vi "RIOduino Periodic.vi"() -> (3 "GearMode":string)   [LabVIEW 2016]
uses:
  TypeDefs/GearCollectState_Type.ctl
  TypeDefs/TurretAimState_Type.ctl
  Global_Var-RefNum/GlobalVar_LED.vi
  <vilib>/Rock Robotics/SystemInterfaces/i2clib/i2c_bus.ctl
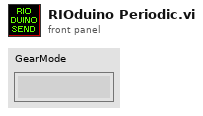
[diagram p1: front panel]
types:
  T1 = typedef "TurretAimState_Type.ctl" = enum16{"Idle", "SearchLeft", "SearchRight", "FindNewTarget", "TargetAcquired"}
  T2 = typedef "GearCollectState_Type.ctl" = enum16{"Store Gear", "Wait For Gear", "Idle"}
  T3 = typedef "i2c_bus.ctl" = enum16{"I2C On-Board", "I2C MXP", "Invalid"}
  T4 = typedef "WPI_I2CDevRef.ctl" = cluster{"DevStatus":errorcluster, "Device Address":u8, "Handle":i32, "I2C Bus":T3}
  T5 = typedef "GearPlaceState_Type.ctl" = enum16{"Idle", "Wait for Peg", "Allign To Lift", "Arm Gear", "Place Gear", "Return to Ready", "Disarm Gear"}
  T6 = typedef "WPI_DriverStationRobotMode2.ctl" = enum16{"Autonomous Disabled", "Autonomous Enabled", "Teleop Disabled", "Teleop Enabled", "Disconnected", "Finish", "Test Disabled", "Test Enabled", "Emergency Stopped"}
  T7 = typedef "WPI_DriverStationAllianceInfo.ctl" = enum16{"Red", "Blue", "Invalid"}
  T8 = typedef "AutoMode_Type.ctl" = enum16{"GearRight", "GearMiddle", "GearLeft", "Shoot&GearMiddle", "BaselineOnly", "Shoot&Baseline"}
  T9 = cluster{u8, u8, u8, u8, u8, u8, u8, "YoYoPosition":u8, "UltraPosition":u8, u8}
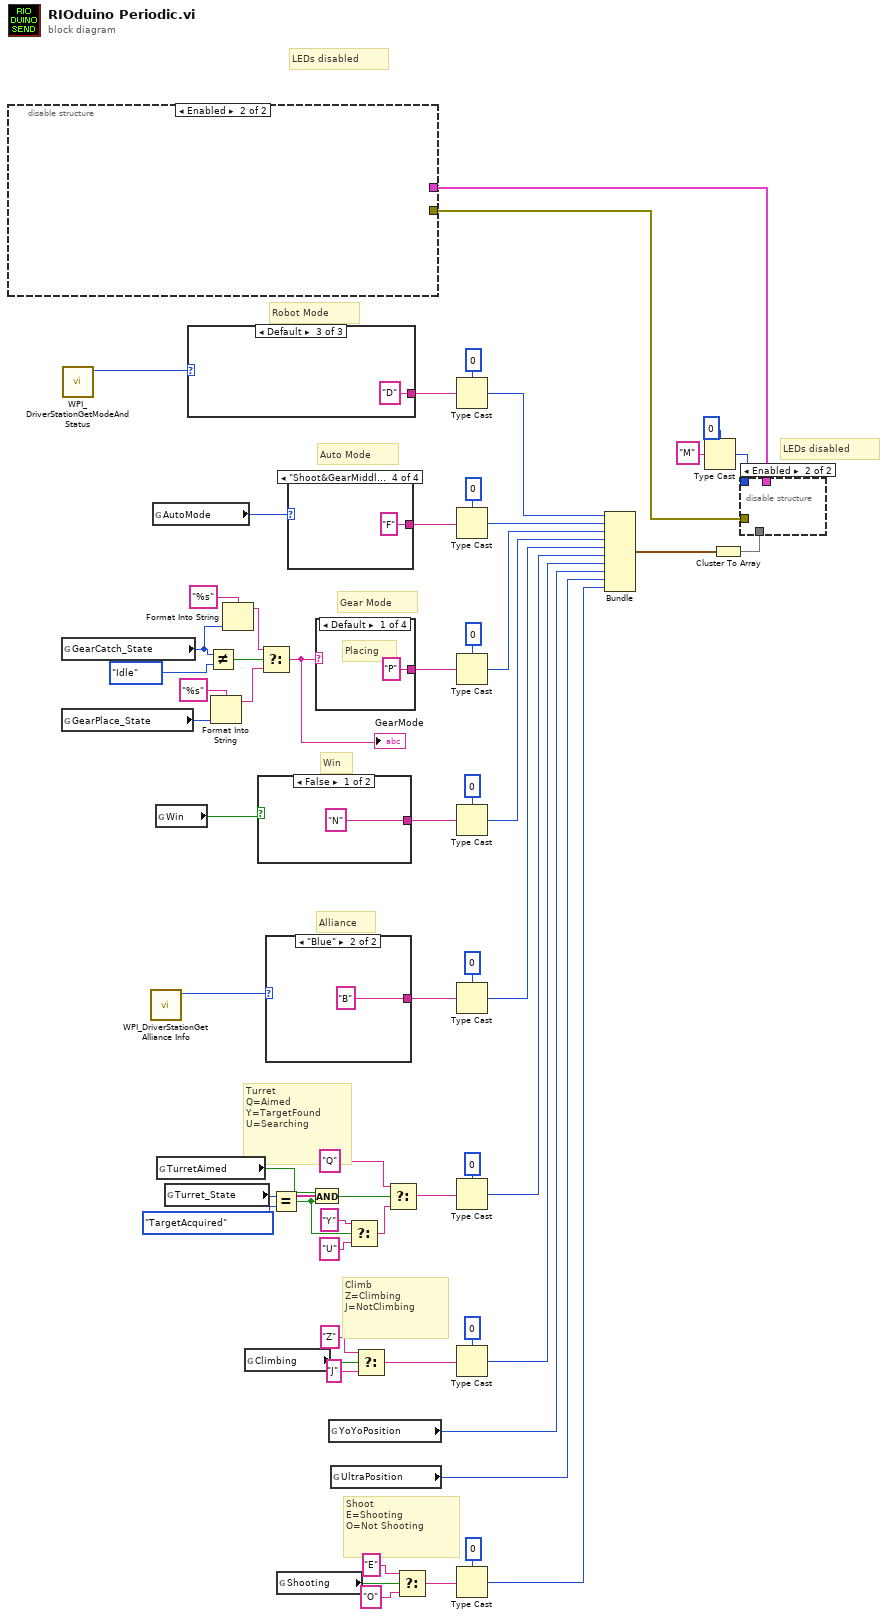
[diagram p0: block diagram]
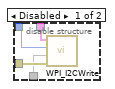
[diagram p2: hidden frame]
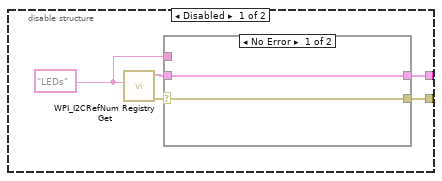
[diagram p3: hidden frame]
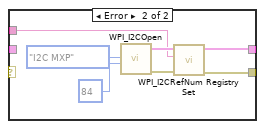
[diagram p4: hidden frame]
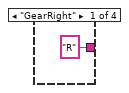
[diagram p5: hidden frame]
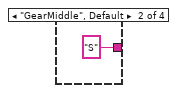
[diagram p6: hidden frame]
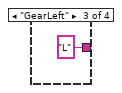
[diagram p7: hidden frame]
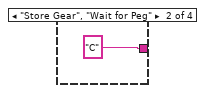
[diagram p8: hidden frame]
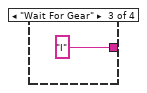
[diagram p9: hidden frame]
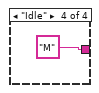
[diagram p10: hidden frame]
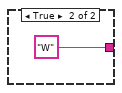
[diagram p11: hidden frame]
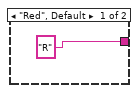
[diagram p12: hidden frame]
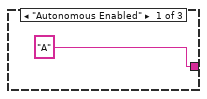
[diagram p13: hidden frame]
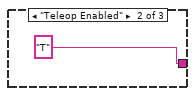
[diagram p14: hidden frame]
diagram:
  # "LEDs disabled"
  # "LEDs disabled"
  # "Shoot\nE=Shooting\nO=Not Shooting"
  # "Climb\nZ=Climbing\nJ=NotClimbing"
  # "Turret\nQ=Aimed\nY=TargetFound\nU=Searching"
  # "Alliance"
  # "Win"
  # "Gear Mode"
  # "Robot Mode"
  # "Auto Mode"
  n1 = disable-structure shown="Enabled" {
    disable-tunnel: [w66 _] -> w61
    disable-tunnel: [w65 _] -> w60
    frame Disabled {
      w64 = "LEDs" ("refnum name")
      n2 = call <vilib>:"WPI_I2CRefNum Registry Get.vi"("refnum name"=w64) -> ("error out"=w62:errorcluster, "I2CDevRef"=w63:T4)  [unwired: 9 in]
      n3 = case shown="No Error" w62 {
        selector: w62 -> [w68 _]
        tunnel: [w68 w70] -> w66
        tunnel: [w67 w71] -> w65
        tunnel: w63 -> [w67 _]
        tunnel: w64 -> [_ w69]
        frame No Error {
        }
        frame Error {
          n4 = call <vilib>:"WPI_I2COpen.vi"("Device Address"=u8 84, "I2C Bus"=i2c_bus."I2C MXP") -> ("error out"=w73:errorcluster, "I2CDevRef"=w72:T4)  [unwired: 8 in]
          n5 = call <vilib>:"WPI_I2CRefNum Registry Set.vi"("error in (no error)"=w73, "refnum name"=w69, "I2CDevRef"=w72) -> ("error out"=w70:errorcluster, "I2CDevRef"=w71:T4)  [unwired: 7 in]
        }
      }
    }
    frame Enabled {
    }
  }
  n6 = global read "GlobalVar_LED.vi" "GearCatch_State"() -> (w37:T2)
  n7 = global read "GlobalVar_LED.vi" "GearPlace_State"() -> (w33:T5)
  n8 = call <vilib>:"WPI_DriverStationGetModeAndStatus.vi"() -> ("Robot Mode"=w40:T6)  [unwired: 10 in, 1 out]
  n9 = call <vilib>:"WPI_DriverStationGet Alliance Info.vi"() -> ("Alliance"=w50:T7)  [unwired: 10 in, 1 out]
  n10 = global read "GlobalVar_LED.vi" "AutoMode"() -> (w2:T8)
  n11 = global read "GlobalVar_LED.vi" "Win"() -> (w30:bool)
  n12 = global read "GlobalVar_LED.vi" "TurretAimed"() -> (w25:bool)
  n13 = global read "GlobalVar_LED.vi" "Turret_State"() -> (w27:T1)
  n14 = case shown="Default" w40 {
    tunnel: ["A" "T" "D"] -> w53
    frame "Autonomous Enabled" {
    }
    frame "Teleop Enabled" {
    }
    frame Default {
    }
  }
  n15 = Not Equal?(x=w37, y=GearCollectState_Type."Idle") -> (x != y?=w38:bool)
  n16 = Format Into String(format string="%s", w33) -> (resulting string=w32:string)  [unwired: 2 in, 1 out]
  n17 = Format Into String(format string="%s", w37) -> (resulting string=w35:string)  [unwired: 2 in, 1 out]
  n18 = global read "GlobalVar_LED.vi" "Climbing"() -> (w16:bool)
  n19 = case shown="False" w30 {
    tunnel: ["N" "W"] -> w43
    frame False {
    }
    frame True {
    }
  }
  n20 = Select(t=w35, s=w38, f=w32) -> (s? t:f=w31:string)
  "GearMode" <- w31
  n21 = case shown="\"Blue\"" w50 {
    tunnel: ["R" "B"] -> w48
    frame "Red", Default {
    }
    frame "Blue" {
    }
  }
  n22 = Equal?(x=w27, y=TurretAimState_Type."TargetAcquired") -> (x = y?=w21:bool)
  n23 = global read "GlobalVar_LED.vi" "Shooting"() -> (w6:bool)
  n24 = case shown="\"Shoot&GearMiddle\"" w2 {
    tunnel: ["R" "S" "L" "F"] -> w1
    frame "GearRight" {
    }
    frame "GearMiddle", Default {
    }
    frame "GearLeft" {
    }
    frame "Shoot&GearMiddle" {
    }
  }
  n25 = And(x=w25, y=w21) -> (x .and. y?=w24:bool)
  n26 = case shown="Default" w31 {
    tunnel: ["P" "C" "I" "M"] -> w41
    frame Default {
      # "Placing"
    }
    frame "Store Gear", "Wait for Peg" {
    }
    frame "Wait For Gear" {
    }
    frame "Idle" {
    }
  }
  n27 = global read "GlobalVar_LED.vi" "YoYoPosition"() -> (w10:u8)
  n28 = global read "GlobalVar_LED.vi" "UltraPosition"() -> (w9:u8)
  n29 = Select(t="Y", s=w21, f="U") -> (s? t:f=w22:string)
  n30 = Select(t="Z" ("f"), s=w16, f="J") -> (s? t:f=w14:string)
  n31 = Select(t="Q", s=w24, f=w22) -> (s? t:f=w18:string)
  n32 = Select(t="E" ("f"), s=w6, f="O") -> (s? t:f=w4:string)
  n33 = Type Cast(type=u8 0, x=w53) -> (*(type *) &x=w52:u8)
  n34 = Type Cast(type=u8 0, x=w1) -> (*(type *) &x=w46:u8)
  n35 = Type Cast(type=u8 0, x=w41) -> (*(type *) &x=w55:u8)
  n36 = Type Cast(type=u8 0, x=w43) -> (*(type *) &x=w44:u8)
  n37 = Type Cast(type=u8 0, x=w48) -> (*(type *) &x=w29:u8)
  n38 = Type Cast(type=u8 0, x=w18) -> (*(type *) &x=w17:u8)
  n39 = Type Cast(type=u8 0, x=w14) -> (*(type *) &x=w11:u8)
  n40 = Type Cast(type=u8 0, x=w4) -> (*(type *) &x=w3:u8)
  n41 = Bundle(w52, w46, w55, w44, w29, w17, w11, "YoYoPosition"=w10, "UltraPosition"=w9, w3) -> (w42:T9)  [unwired: 1 in]
  n42 = Type Cast(type=u8 0, x="M") -> (*(type *) &x=w57:u8)
  n43 = Cluster To Array(cluster=w42) -> (array=w51:u8[])
  n44 = disable-structure shown="Enabled" {
    disable-tunnel: w61 -> [w94 _]
    disable-tunnel: w60 -> [w93 _]
    disable-tunnel: w57 -> [w92 _]
    disable-tunnel: w51 -> [w91 _]
    frame Disabled {
      n45 = call <vilib>:"WPI_I2CWrite.vi"("error in (no error)"=w94, "I2CDataToSend"=w91, "I2CRegister"=w92, "I2CDevRef"=w93) -> ()  [unwired: 6 in, 2 out]
    }
    frame Enabled {
    }
  }
